vi "05_ServiceByteParsing.vi"(11 "InputByte":u8) -> (0 "Range":bool, 1 "LED2":bool, 2 "LED1":bool, 3 "TrigState":bool)   [LabVIEW 2017]
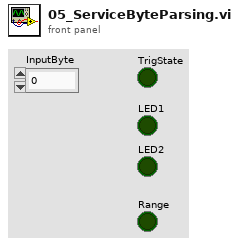
[diagram p1: front panel]
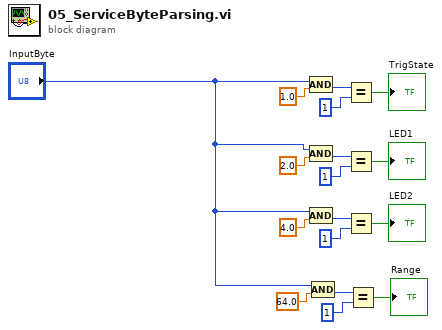
[diagram p0: block diagram]
diagram:
  n1 = Compound Arithmetic op=AND("InputByte", 1.0 ("value")) -> (w17:i32)
  n2 = Compound Arithmetic op=AND("InputByte", 2.0 ("value")) -> (w14:i32)
  n3 = Compound Arithmetic op=AND("InputByte", 4.0 ("value")) -> (w11:i32)
  n4 = Compound Arithmetic op=AND("InputByte", 64.0 ("value")) -> (w8:i32)
  n5 = Equal?(x=w17, y=1) -> (x = y?=→"TrigState":bool)
  n6 = Equal?(x=w14, y=1) -> (x = y?=→"LED1":bool)
  n7 = Equal?(x=w11, y=1) -> (x = y?=→"LED2":bool)
  n8 = Equal?(x=w8, y=1) -> (x = y?=→"Range":bool)
